vi "单个流程写入.vi"(5 "简易流程Id":u16(ring), 6 "是否是简易流程":bool, 7 "添加的路径":path, 8 "error in (no error)":errorcluster caption="错误输入（无错误）", 9 "量程":enum16{"低量程", "高量程"}(ring), 10 "测量模式":T1(ring), 11 "测量参数":u16(ring) items=["总氮"=2, "总磷"=1, "氨氮"=3, "COD"=22]) -> (0 "error out":errorcluster caption="错误输出", 3 "步数":i32)   [LabVIEW 2016, in "斯坦道CODCr.lvlib"]
panel:
  out "数组 2":u16[][](array[numeric]) format="0x%04x"
  out "大小":i32
  out "交织的数组":u16[](array[numeric]) format="0x%04x"
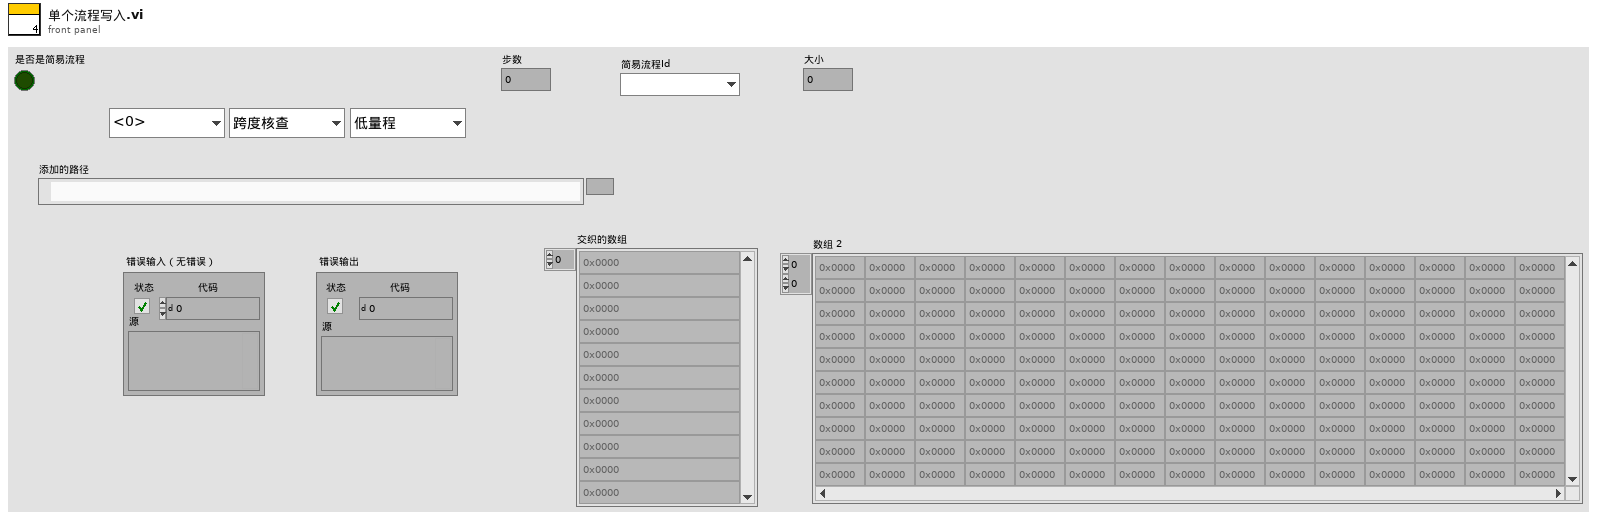
[diagram p1: front panel]
types:
  T1 = enum16{"跨度核查", "水样测量", "零点核查", "标样核查", "加标回收", "快捷测试", "空白校准", "标样校准"}
  T2 = cluster{"测量参数":u16, "测量模式":enum16{"跨度核查", "水样测量", "零点核查", "标样核查", "加标回收", "快捷测试", "空白校准", "标样校准"}, u16}
  T3 = cluster{"port":u32, "dac":u8, "adc":u8, "time":u16, "步骤名":string}[]
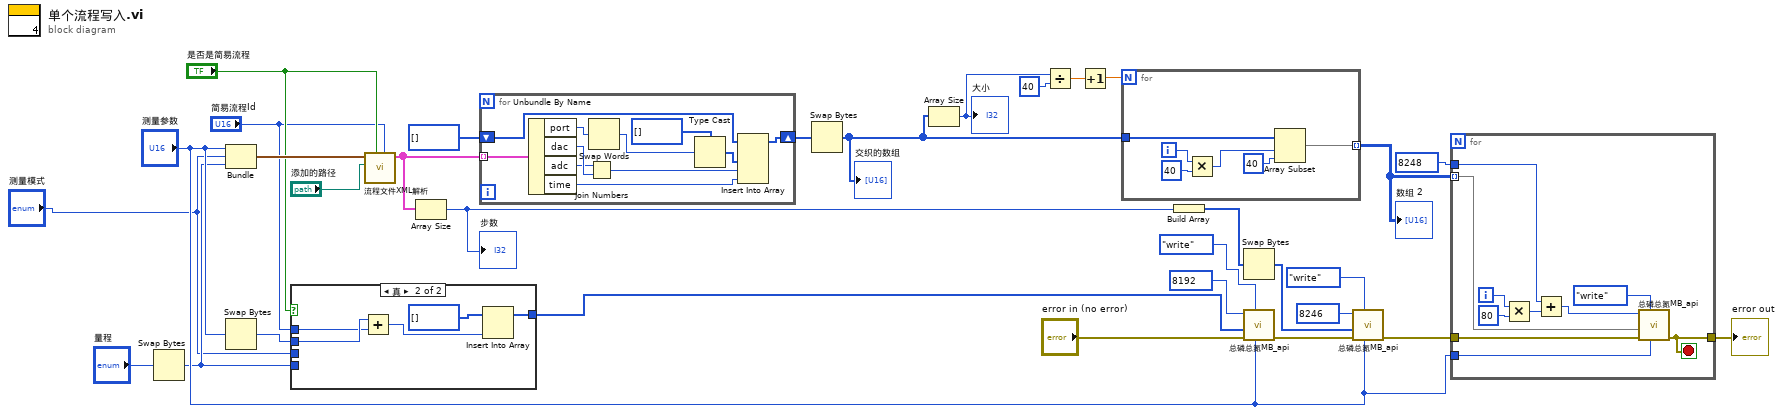
[diagram p0: block diagram]
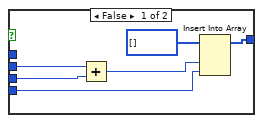
[diagram p2: hidden frame]
diagram:
  n1 = Swap Bytes(anything="量程") -> (byte swapped=w4:u16)
  n2 = Bundle("测量参数"="测量参数", "测量模式"="测量模式", w4) -> (w21:T2)  [unwired: 1 in]
  n3 = Swap Bytes(anything="测量参数") -> (byte swapped=w6:u16)
  n4 = case shown="真" "是否是简易流程" {
    tunnel: [w35 w40] -> w25
    tunnel: "测量模式" -> [w34 _]
    tunnel: w6 -> [w33 w39]
    tunnel: w4 -> [w32 _]
    tunnel: "简易流程Id" -> [_ w38]
    frame False {
      n5 = Add(x=w33, y=w34) -> (x+y=w37:u16)
      n6 = Insert Into Array(array=u16[] [] ("数组"), new element #1=w37, new element #2=w32) -> (w35:u16[])  [unwired: 1 in]
    }
    frame True {
      n7 = Add(x=w39, y=w38) -> (x+y=w42:u16)
      n8 = Insert Into Array(array=u16[] [] ("数组"), new element=w42) -> (w40:u16[])  [unwired: 1 in]
    }
  }
  n9 = call "流程文件XML解析.vi"("简易流程Id"="简易流程Id", "是否是简易流程"="是否是简易流程", "添加的路径"="添加的路径", "参数簇"=w21) -> ("数组"=w13:T3)  [unwired: 7 in]
  n10 = Array Size(array=w13) -> (size(s)=w8:i32)
  "步数" <- w8
  n11 = for {
    tunnel: w13 -> [w53] mode=indexing
    shift-right: [w48] -> w18
    shift-left: u16[] [] -> [w46]
    n12 = Unbundle By Name(w53) -> ("port"=w51:u32, "dac"=w44:u8, "adc"=w43:u8, "time"=w49:u16)
    n13 = Join Numbers(hi=w43, lo=w44) -> ((hi.lo)=w50:u16)
    n14 = Swap Words(1:w51) -> (0:w45:u32)
    n15 = Type Cast(type=u16[] [], x=w45) -> (*(type *) &x=w47:u16[])
    n16 = Insert Into Array(array=w46, new element #1=w47, new element #2=w50, new element #3=w49) -> (w48:u16[])  [unwired: 1 in]
  }
  n17 = Swap Bytes(anything=w18) -> (byte swapped=w15:u16[])
  "交织的数组" <- w15
  n18 = Array Size(array=w15) -> (size(s)=w17:i32)
  "大小" <- w17
  n19 = Divide(x=w17, y=40) -> (x/y=w11:dbl)
  n20 = Increment(x=w11) -> (x+1=w10:dbl)
  n21 = for {
    N: w10 -> [_]
    tunnel: w15 -> [w57]
    tunnel: [w54] -> w14 mode=indexing
    i -> [w59]
    n22 = Multiply(x=w59, y=40) -> (x*y=w56:i32)
    n23 = Array Subset(array=w57, index=w56, length=40 ("y")) -> (w54:u16[])
  }
  "数组 2" <- w14
  n24 = Build Array(w8) -> (w12:i32[])
  n25 = Swap Bytes(anything=w12) -> (byte swapped=w9:i32[])
  n26 = call "总磷总氮MB_api.vi"("Slave ID"="测量参数", "STEP"=enum16{"open", "read", "write", "close"}."write", "Error in"="error in (no error)", "values"=w25, "starting address"=u16 8192) -> ("error out"=w28:errorcluster)  [unwired: 4 in, 2 out]
  n27 = call "总磷总氮MB_api.vi"("Slave ID"="测量参数", "STEP"=enum16{"open", "read", "write", "close"}."write", "Error in"=w28, "values"=w9, "starting address"=u16 8246) -> ("error out"=w24:errorcluster)  [unwired: 4 in, 2 out]
  n28 = for {
    tunnel: u16 8248 ("starting address") -> [w63]
    tunnel: w24 -> [w69]
    tunnel: [w67] -> w22
    tunnel: "测量参数" -> [w66]
    tunnel: w14 -> [w65] mode=indexing
    i -> [w62]
    stop <- w67 stop-if-true
    n29 = Multiply(x=w62, y=80) -> (x*y=w61:i32)
    n30 = Add(x=w63, y=w61) -> (x+y=w64:i32)
    n31 = call "总磷总氮MB_api.vi"("Slave ID"=w66, "STEP"=enum16{"open", "read", "write", "close"}."write", "Error in"=w69, "values"=w65, "starting address"=w64) -> ("error out"=w67:errorcluster)  [unwired: 4 in, 2 out]
  }
  "error out" <- w22
